vi "test_Bitfile Reload_Scalar Data Type Change SGL.vi"(8 "error in (no error)":errorcluster, 11 "TestCase in":refnum<class "Bitfile Reload System Tests.lvclass">) -> (0 "error out":errorcluster, 3 "TestCase out":refnum<class "Bitfile Reload System Tests.lvclass">)   [LabVIEW 2020, in "Bitfile Reload System Tests.lvclass"]
uses:
  Bitfile Reload System Tests.lvclass
  C:/Users/Administrator/Desktop/GIT/niveristand-custom-device-testing-tools/VeriStandTestCase/VeriStandTestCase.lvclass
  APIs/Scripting API/TypeDefs/Output Scalar Data.ctl
  Addon/Addon Shared/Types/FPGA Addon Data Type.ctl
  <vilib>/NI VeriStand/Execution/Workspace/NI VeriStand - Get Single Channel Value.vi
  <vilib>/addons/_JKI Toolkits/VI Tester/TestCase.llb/TestCase.lvclass
  FPGA Addon Test Class/FPGA Addon Test Class.lvclass
  <vilib>/NI VeriStand/Execution/Workspace/NI_VS Workspace ExecutionAPI.lvlib
  Addon/Addon System Explorer/FPGA Addon System Explorer.lvlib
  APIs/Scripting API/Scripting API.lvlib
  Addon/Addon Shared/FPGA Addon Shared.lvlib
  C:/Program Files (x86)/National Instruments/LabVIEW 2020/vi.lib/addons/_JKI Toolkits/VI Tester/TestCase.llb/TestCase.lvclass
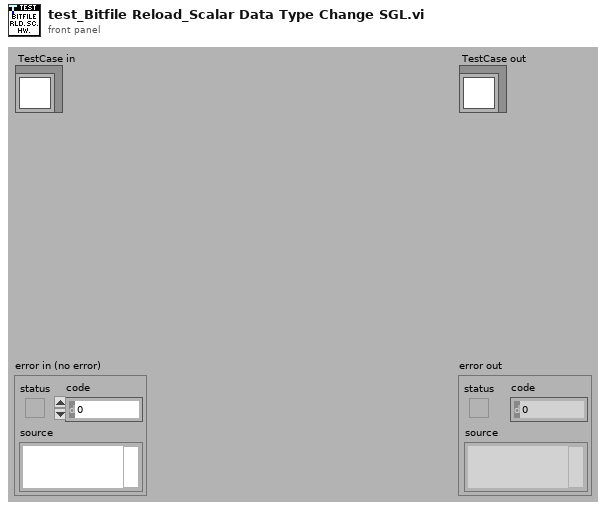
[diagram p1: front panel]
types:
  T1 = typedef "Scripting API.lvlib/Output Scalar Data.ctl" = cluster{"Bitfile Name":string, "SysDef Channel Name":string, "Imported":bool, "Data Type":T2}
  T2 = typedef "FPGA Addon Shared.lvlib/FPGA Addon Data Type.ctl" = enum8{"<Null>", "I8", "I16", "I32", "I64", "U8", "U16", "U32", "U64", "SGL", "Boolean", "Analog PWM In Settings", "Analog PWM In", "Digital PWM In Settings", "Digital PWM In", "Digital PWM Out", "Sine Out", "FXP", "FXP+/-24.5", "FXP+/-16.5", "FXP+/-32.8", "FXP+/-64.32", "FXP+/-16.7", "FXP+/-20.5", "FXP+/-27.5", "FXP+/-32.16", "FXP+16.3", "FXP+18.3", "Digital Static In", "Digital Static Out", "Digital Static In Settings", "Digital WSS Out", "Quad Encoder Settings", "Quad Encoder In", "Group"}
  T3 = typedef "Custom Device API.lvlib/Custom Device Item Ref.ctl" = u64
  T4 = typedef "NI_VS Workspace ExecutionAPI.lvlib/WorkspaceAPI.ctl" = refnum<k24>
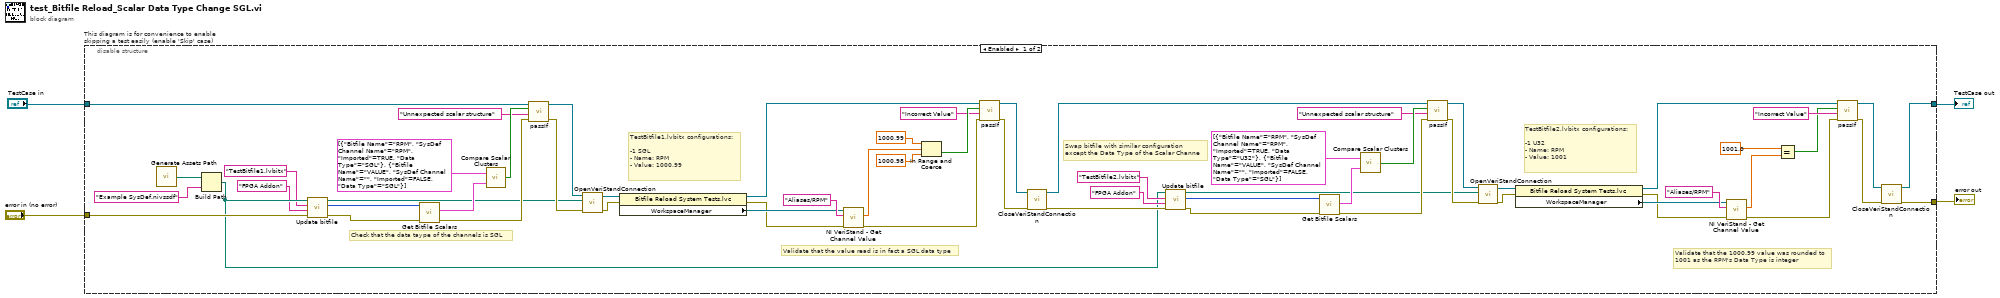
[diagram p0: block diagram]
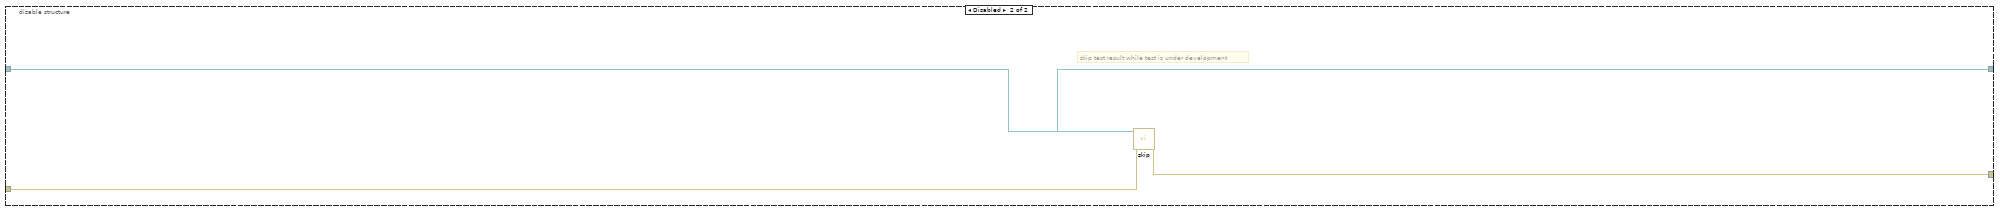
[diagram p2: hidden frame]
diagram:
  n1 = disable-structure "This diagram is for convenience to enable skipping a test easily (enable 'Skip' case)" shown="Enabled" {
    disable-tunnel: "TestCase in" -> [w28 w68]
    disable-tunnel: [w33 w66] -> w1
    disable-tunnel: [w15 w67] -> w3
    disable-tunnel: "error in (no error)" -> [w14 w65]
    frame Enabled {
      # "Check that the data taype of the channels is SGL"
      # "Validate that the 1000.99 value was rounded to\n1001 as the RPM's Data Type is integer"
      # "Swap bitfile with similar configuration\nexcept the Data Type of the Scalar Channe"
      # "Validate that the value read is in fact a SGL data type"
      # "TestBitfile2.lvbitx configurations:\n\n-1 U32\n- Name: RPM\n- Value: 1001"
      # "TestBitfile1.lvbitx configurations:\n\n-1 SGL\n- Name: RPM\n- Value: 1000.99"
      n2 = call "Generate Assets Path.vi"() -> ("Assets path"=w63:path)
      n3 = Build Path(base path=w63, name or relative path="Example SysDef.nivssdf") -> (appended path=w13:path)
      n4 = call "Update bitfile.vi"("error in (no error)"=w14, "FPGA addon name"="FPGA Addon", "bitfile name"="TestBitfile1.lvbitx", "sysdef path in"=w13) -> ("error out"=w11:errorcluster, "FPGA addon refnum out"=w10:T3, "sysdef path out"=w12:path)  [unwired: 5 in]
      n5 = call "Get Bitfile Scalars.vi"("error in"=w11, "FPGA addon refnum in"=w10) -> ("error out"=w27:errorcluster, "bitfile scalars out"=w30:T1[])  [unwired: 7 in, 1 out]
      n6 = call "Compare Scalar Clusters.vi"("Target bitfile scalars in"=w30, "Reference bitfile scalars in"=T1[] [{"Bitfile Name"="RPM", "SysDef Channel Name"="RPM", "Imported"=TRUE, "Data Type"=enum."SGL"}, {"Bitfile Name"="VALUE", "SysDef Channel Name"="", "Imported"=FALSE, "Data Type"=enum."SGL"}] ("bitfile scalars out")) -> ("Equal ?"=w26:bool)
      n7 = call-dynamic "passIf.vi"("error in (no error)"=w27, "message (\"\")"="Unnexpected scalar structure" ("message (\"\")"), "pass"=w26, "TestCase in"=w28) -> ("error out"=w24:errorcluster, "TestCase out"=w29:refnum<class "Bitfile Reload System Tests.lvclass">)  [unwired: 6 in]
      n8 = call-dynamic "OpenVeriStandConnection.vi"("error in (no error)"=w24, "System Definition File"=w12, "VeriStand Test Case in"=w29) -> ("error out"=w49:errorcluster, "VeriStand Test Case out"=w48:refnum<class "Bitfile Reload System Tests.lvclass">)  [unwired: 6 in, 1 out]
      n9 = property class="Bitfile Reload System Tests.lvc"(reference=w48, error in=w49) -> (reference out=w54:refnum<class "Bitfile Reload System Tests.lvclass">, error out=w50:errorcluster, "WorkspaceManager"=w51:T4)
      n10 = call-poly <vilib>:"NI VeriStand - Get Channel Value.vi"("error in (no error)"=w50, "Channel"="Aliases/RPM", "WorkspaceManager in"=w51) -> ("error out"=w53:errorcluster, "Value"=w32:dbl)  [unwired: 6 in, 1 out]
      n11 = In Range and Coerce(upper limit=1000.99, x=w32, lower limit=1000.98) -> (In Range?=w58:bool)  [unwired: 1 out]
      n12 = call-dynamic "passIf.vi"("error in (no error)"=w53, "message (\"\")"="Incorrect Value" ("message (\"\")"), "pass"=w58, "TestCase in"=w54) -> ("error out"=w59:errorcluster, "TestCase out"=w60:refnum<class "Bitfile Reload System Tests.lvclass">)  [unwired: 6 in]
      n13 = call-dynamic "CloseVeriStandConnection.vi"("error in (no error)"=w59, "VeriStand Test Case in"=w60) -> ("error out"=w47:errorcluster, "VeriStand Test Case out"=w23:refnum<class "Bitfile Reload System Tests.lvclass">)  [unwired: 8 in]
      n14 = call "Update bitfile.vi"("error in (no error)"=w47, "FPGA addon name"="FPGA Addon", "bitfile name"="TestBitfile2.lvbitx", "sysdef path in"=w13) -> ("error out"=w7:errorcluster, "FPGA addon refnum out"=w9:T3, "sysdef path out"=w8:path)  [unwired: 5 in]
      n15 = call "Get Bitfile Scalars.vi"("error in"=w7, "FPGA addon refnum in"=w9) -> ("error out"=w18:errorcluster, "bitfile scalars out"=w20:T1[])  [unwired: 7 in, 1 out]
      n16 = call "Compare Scalar Clusters.vi"("Target bitfile scalars in"=w20, "Reference bitfile scalars in"=T1[] [{"Bitfile Name"="RPM", "SysDef Channel Name"="RPM", "Imported"=TRUE, "Data Type"=enum."U32"}, {"Bitfile Name"="VALUE", "SysDef Channel Name"="", "Imported"=FALSE, "Data Type"=enum."SGL"}] ("bitfile scalars out")) -> ("Equal ?"=w17:bool)
      n17 = call-dynamic "passIf.vi"("error in (no error)"=w18, "message (\"\")"="Unnexpected scalar structure" ("message (\"\")"), "pass"=w17, "TestCase in"=w23) -> ("error out"=w21:errorcluster, "TestCase out"=w22:refnum<class "Bitfile Reload System Tests.lvclass">)  [unwired: 6 in]
      n18 = call-dynamic "OpenVeriStandConnection.vi"("error in (no error)"=w21, "System Definition File"=w8, "VeriStand Test Case in"=w22) -> ("error out"=w38:errorcluster, "VeriStand Test Case out"=w37:refnum<class "Bitfile Reload System Tests.lvclass">)  [unwired: 6 in, 1 out]
      n19 = property class="Bitfile Reload System Tests.lvc"(reference=w37, error in=w38) -> (reference out=w43:refnum<class "Bitfile Reload System Tests.lvclass">, error out=w39:errorcluster, "WorkspaceManager"=w40:T4)
      n20 = call-poly <vilib>:"NI VeriStand - Get Channel Value.vi"("error in (no error)"=w39, "Channel"="Aliases/RPM", "WorkspaceManager in"=w40) -> ("error out"=w42:errorcluster, "Value"=w36:dbl)  [unwired: 6 in, 1 out]
      n21 = Equal?(x=1001.0, y=w36) -> (x = y?=w34:bool)
      n22 = call-dynamic "passIf.vi"("error in (no error)"=w42, "message (\"\")"="Incorrect Value" ("message (\"\")"), "pass"=w34, "TestCase in"=w43) -> ("error out"=w45:errorcluster, "TestCase out"=w46:refnum<class "Bitfile Reload System Tests.lvclass">)  [unwired: 6 in]
      n23 = call-dynamic "CloseVeriStandConnection.vi"("error in (no error)"=w45, "VeriStand Test Case in"=w46) -> ("error out"=w15:errorcluster, "VeriStand Test Case out"=w33:refnum<class "Bitfile Reload System Tests.lvclass">)  [unwired: 8 in]
      n24 = call "Reload Bitfile.vi"() -> ()  [unwired: 10 in, 2 out]
    }
    frame Disabled {
      # "skip test result while test is under development"
      n25 = call <vilib>:"skip.vi"("error in (no error)"=w65, "TestCase in"=w68) -> ("error out"=w67:errorcluster, "TestCase out"=w66:refnum<class "Bitfile Reload System Tests.lvclass">)  [unwired: 8 in]
    }
  }
  "error out" <- w3
  "TestCase out" <- w1
